vi "Nfocus driver V0.4.vi"(5 "error in":errorcluster, 8 "Refs In":T1) -> (0 "error out":errorcluster)   [LabVIEW 2016]
panel:
  out "Running":bool
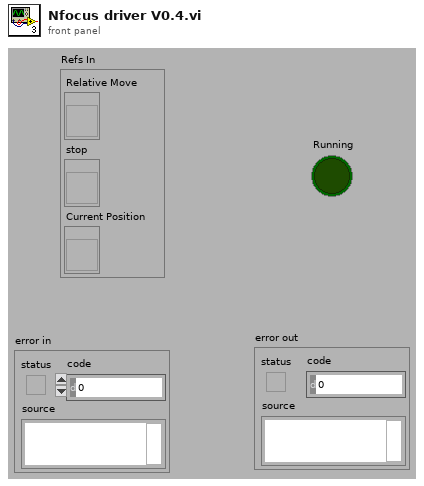
[diagram p1: front panel]
types:
  T1 = cluster{"Relative Move":refnum<vi>, "stop":refnum<vi>, "Current Position":refnum<vi>}
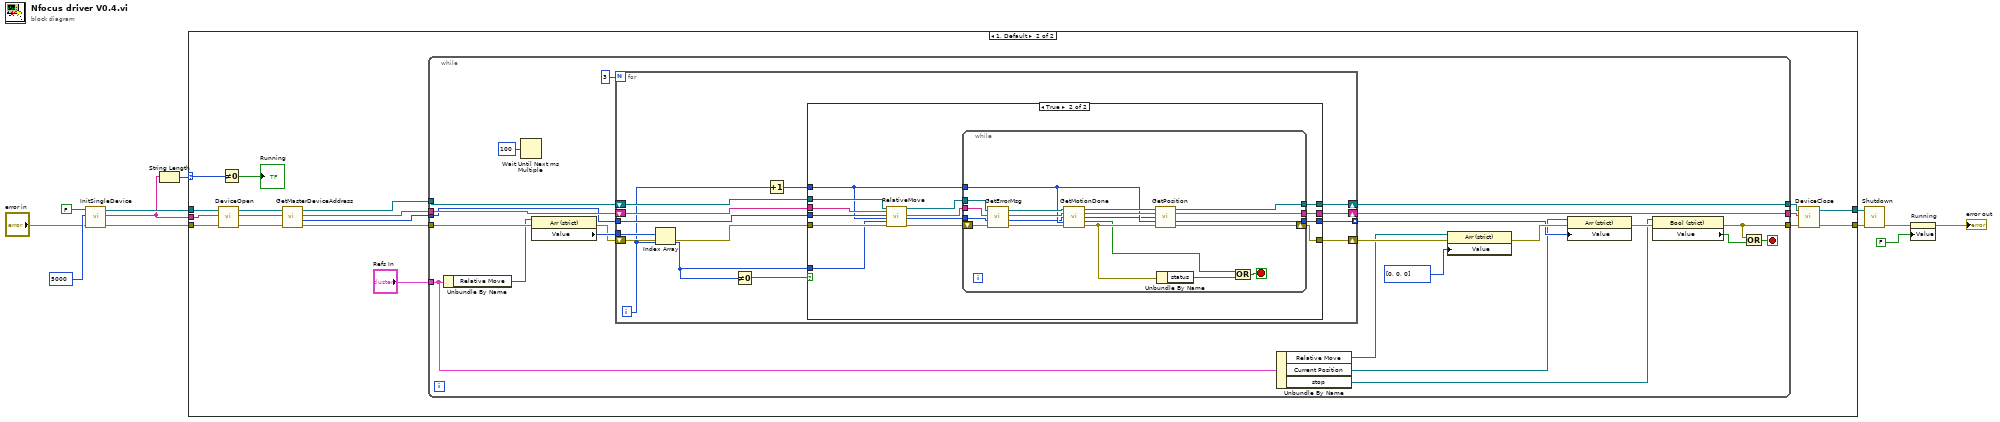
[diagram p0: block diagram]
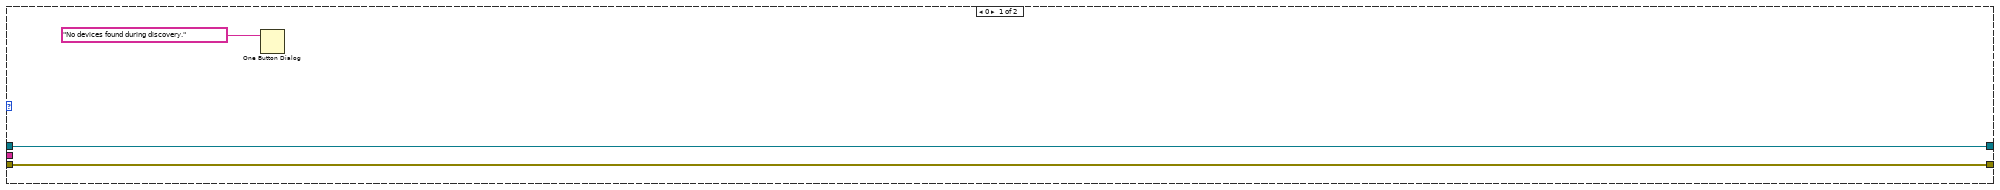
[diagram p2: hidden frame]
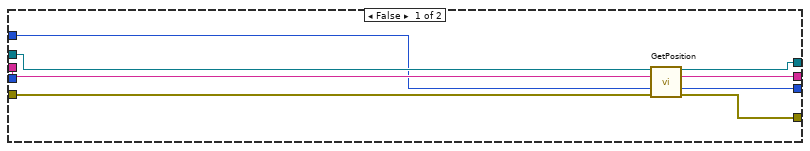
[diagram p3: hidden frame]
diagram:
  n1 = call "InitSingleDevice.vi"("error in (no error)"="error in", "msecDelayForDiscovery"=5000, "logging"=FALSE) -> ("error out"=w5:errorcluster, "DeviceKey Out"=w6:string, "CmdLib Out"=w8:refnum<k24>)  [unwired: 2 in]
  n2 = String Length(string=w6) -> (length=w7:i32)
  n3 = case shown="1, Default" w7 {
    selector: w7 -> [_ w18]
    tunnel: [w14 w20] -> w10
    tunnel: [w13 w22] -> w9
    tunnel: w8 -> [w14 w26]
    tunnel: w6 -> [_ w28]
    tunnel: w5 -> [w13 w30]
    frame 0 {
      n4 = One Button Dialog(message="No devices found during discovery.") -> ()  [unwired: 1 in, 1 out]
    }
    frame 1, Default {
      n5 = call "DeviceOpen.vi"("error in (no error)"=w30, "DeviceKey In"=w28, "CmdLib In"=w26) -> ("error out"=w29:errorcluster, "DeviceKey Out"=w27:string, "CmdLib Out"=w25:refnum<k24>)  [unwired: 2 in]
      n6 = Not Equal To 0?(x=w18) -> (x != 0?=→"Running":bool)
      n7 = call "GetMasterDeviceAddress.vi"("error in (no error)"=w29, "DeviceKey In"=w27, "CmdLib In"=w25) -> ("error out"=w19:errorcluster, "Device Address"=w33:i32, "DeviceKey Out"=w31:string, "CmdLib Out"=w32:refnum<k24>)  [unwired: 1 in]
      n8 = while {
        tunnel: w33 -> [w46]
        tunnel: w32 -> [w48]
        tunnel: [w55] -> w21
        tunnel: w19 -> [w50]
        tunnel: [w53] -> w23
        tunnel: w31 -> [w47]
        tunnel: [w56] -> w24
        tunnel: "Refs In" -> [w39]
        stop <- w54 stop-if-true
        n9 = Unbundle By Name(w39) -> ("Relative Move"=w44:refnum<vi>)
        n10 = Wait Until Next ms Multiple(millisecond multiple=u32 100) -> ()  [unwired: 1 out]
        n11 = property class="Arr (strict)"(reference=w44, error in=w50) -> (error out=w49:errorcluster, "Value"=w51:i32[])  [unwired: 1 out]
        n12 = for {
          N: 3 -> [_]
          tunnel: w51 -> [w66]
          shift-right: [w61] -> w45
          shift-left: w49 -> [w65]
          shift-right: [w68] -> w55
          shift-left: w48 -> [w64]
          shift-right: [w69] -> w56
          shift-left: w47 -> [w63]
          tunnel: w46 -> [w62]
          tunnel: [w60] -> w40 mode=indexing
          i -> [w58]
          n13 = Index Array(array=w66, index=w58) -> (element=w59:i32)
          n14 = Not Equal To 0?(x=w59) -> (x != 0?=w67:bool)
          n15 = Increment(x=w58) -> (x+1=w57:i32)
          n16 = case shown="True" w67 {
            tunnel: w62 -> [_ w91]
            tunnel: w64 -> [w77 w90]
            tunnel: w63 -> [w76 w89]
            tunnel: [w73 w88] -> w69
            tunnel: [w72 w87] -> w68
            tunnel: w65 -> [w75 w86]
            tunnel: [w74 w85] -> w61
            tunnel: [w71 w80] -> w60
            tunnel: w59 -> [_ w79]
            tunnel: w57 -> [w70 w78]
            frame False {
              n17 = call "GetPosition.vi"("CmdLib In"=w77, "DeviceKey In"=w76, "Motor"=w70, "error in (no error)"=w75) -> ("CmdLib Out"=w72:refnum<k24>, "DeviceKey Out"=w73:string, "Position"=w71:i32, "error out"=w74:errorcluster)  [unwired: 7 in, 1 out]
            }
            frame True {
              n18 = call "RelativeMove.vi"("CmdLib In"=w90, "DeviceKey In"=w89, "Device Address In"=w91, "Motor"=w78, "Relative Steps"=w79, "error in (no error)"=w86) -> ("CmdLib Out"=w84:refnum<k24>, "DeviceKey Out"=w83:string, "Device Address Out"=w81:i32, "error out"=w82:errorcluster)  [unwired: 10 in]
              n19 = while {
                tunnel: w78 -> [w107]
                tunnel: w84 -> [w106]
                tunnel: w83 -> [w105]
                tunnel: [w100] -> w87
                tunnel: w81 -> [w99]
                shift-right: [w101] -> w85
                shift-left: w82 -> [w104]
                tunnel: [w96] -> w88
                tunnel: [w92] -> w80
                stop <- w95 stop-if-true
                n20 = call "GetErrorMsg.vi"("error in (no error)"=w104, "Device Address In"=w99, "DeviceKey In"=w105, "CmdLib In"=w106) -> ("error out"=w103:errorcluster, "Device Address Out"=w98:i32, "DeviceKey Out"=w109:string, "CmdLib Out"=w108:refnum<k24>)
                n21 = call "GetMotionDone.vi"("CmdLib In"=w108, "DeviceKey In"=w109, "Device Address In"=w98, "Motor"=w107, "error in (no error)"=w103) -> ("CmdLib Out"=w110:refnum<k24>, "DeviceKey Out"=w111:string, "Device Address Out"=w97:i32, "Is Motion Done"=w94:bool, "error out"=w102:errorcluster)  [unwired: 6 in]
                n22 = call "GetPosition.vi"("CmdLib In"=w110, "DeviceKey In"=w111, "Device Address In"=w97, "Motor"=w107, "error in (no error)"=w102) -> ("CmdLib Out"=w100:refnum<k24>, "DeviceKey Out"=w96:string, "Position"=w92:i32, "error out"=w101:errorcluster)  [unwired: 6 in, 1 out]
                n23 = Unbundle By Name(w102) -> ("status"=w93:bool)
                n24 = Compound Arithmetic op=OR(w94, w93) -> (w95:bool)
              }
            }
          }
        }
        n25 = Unbundle By Name(w39) -> ("Relative Move"=w35:refnum<vi>, "Current Position"=w38:refnum<vi>, "stop"=w37:refnum<vi>)
        n26 = property class="Arr (strict)"(reference=w35, error in=w45, "Value"=i32[] [0, 0, 0]) -> (error out=w42:errorcluster)  [unwired: 1 out]
        n27 = property class="Arr (strict)"(reference=w38, error in=w42, "Value"=w40) -> (error out=w41:errorcluster)  [unwired: 1 out]
        n28 = property on="Property Node" class="Bool (strict)"(reference=w37, error in=w41) -> (error out=w53:errorcluster, "Value"=w52:bool)  [unwired: 1 out]
        n29 = Compound Arithmetic op=OR(w53, w52) -> (w54:bool)
      }
      n30 = call "DeviceClose.vi"("error in (no error)"=w23, "DeviceKey In"=w24, "CmdLib In"=w21) -> ("error out"=w22:errorcluster, "CmdLib Out"=w20:refnum<k24>)  [unwired: 2 in, 1 out]
    }
  }
  n31 = call "Shutdown.vi"("error in (no error)"=w9, "CmdLib In"=w10) -> ("error out"=w3:errorcluster)  [unwired: 4 in, 1 out]
  n32 = property on="Running" class="Bool (strict)"(error in=w3, "Value"=FALSE ("Boolean")) -> (error out=→"error out":errorcluster)  [unwired: 1 in, 1 out]
